vi "Simulate Waveform in Graph (Using DAC).vi"() -> ()   [LabVIEW 2020]
uses:
  <vilib>/DAQmx/read.llb/DAQmx Read (Analog 1D DBL 1Chan NSamp).vi
  <vilib>/DAQmx/create/channels.llb/DAQmx Create Channel (AI-Voltage-Basic).vi
  <vilib>/DAQmx/miscellaneous.llb/DAQmx Fill In Error Info.vi
panel:
  out "error out":errorcluster
  out "Waveform Graph":waveform(dbl)(graph)
  in  "stop":bool
  # "Simulate Waveform in Graph (Using DAC)"
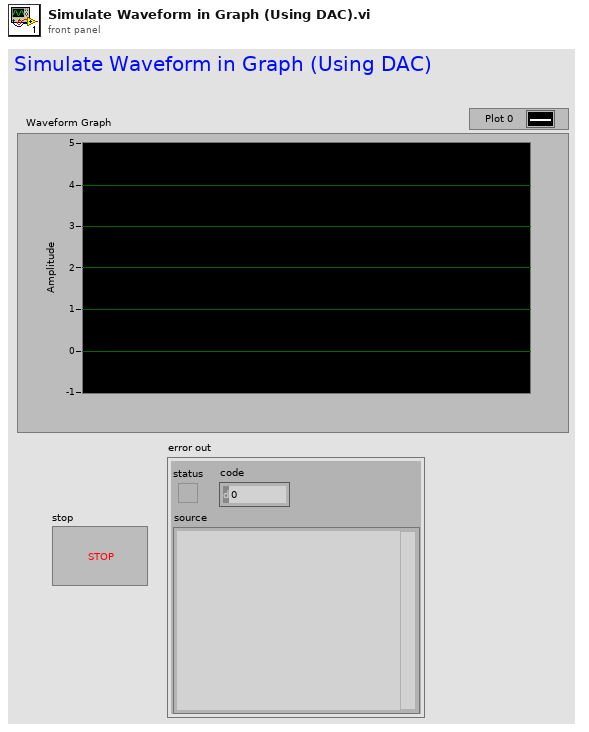
[diagram p1: front panel]
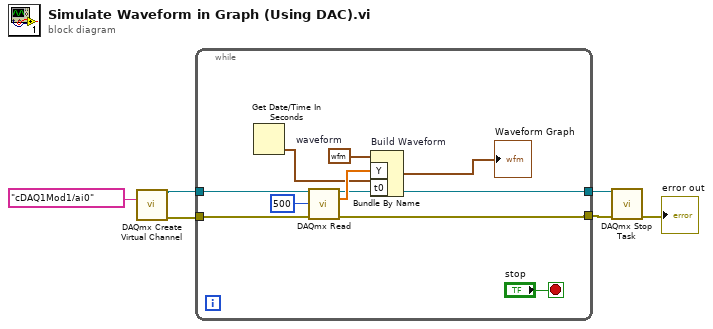
[diagram p0: block diagram]
diagram:
  n1 = call-poly <vilib>:"DAQmx Create Virtual Channel.vi"("physical channels"=tag "cDAQ1Mod1/ai0") -> ("task out"=w5:refnum<k21>, "error out"=w2:errorcluster)  [unwired: 13 in]
  n2 = while {
    tunnel: w5 -> [w12]
    tunnel: w2 -> [w11]
    tunnel: [w10] -> w4
    tunnel: [w9] -> w3
    stop <- "stop" stop-if-true
    w14 = waveform(dbl) {"t0"=timestamp(0 s since 1904-01-01), "dt"=1.0, "Y"=[]}  # waveform
    n3 = Get Date/Time In Seconds() -> (seconds since 1Jan1904=w7:timestamp)
    n4 = call-poly <vilib>:"DAQmx Read.vi"("task/channels in"=w12, "number of samples per channel"=500, "error in"=w11) -> ("task out"=w10:refnum<k21>, "data"=w16:dbl[], "error out"=w9:errorcluster)  [unwired: 10 in]
    n5 = Bundle By Name "Build Waveform"(cluster=w14, "Y"=w16, "t0"=w7) -> (→"Waveform Graph":waveform(dbl))
  }
  n6 = call <vilib>:"DAQmx Stop Task.vi"("task/channels in"=w4, "error in"=w3) -> ("error out"=→"error out":errorcluster)  [unwired: 12 in, 1 out]
